vi "Find Invalid Plugin Groups by ID.vi"(8 "error in (no error)":errorcluster, 10 "plugin ID":string, 11 "Configuration Session in":refnum<class "Configuration Session.lvclass">) -> (0 "error out":errorcluster, 1 "Invalid Groups":string[](array[string]), 3 "Configuration Session out":refnum<class "Configuration Session.lvclass">, 4 "found?":bool)   [LabVIEW 2017, in "DSF Core.lvlib" / "Configuration Session.lvclass"]
uses:
  Configuration Session.lvclass
  Read Plugin Group IDs.vi
  Read All Group IDs.vi
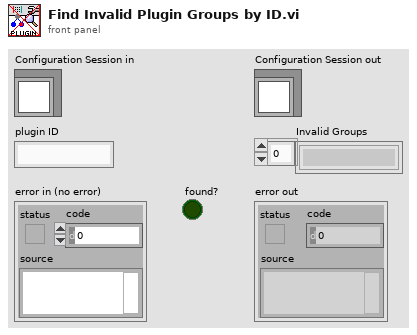
[diagram p1: front panel]
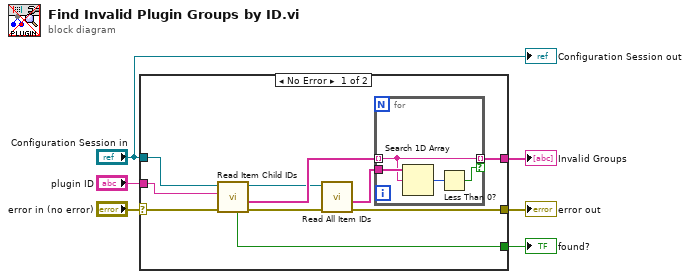
[diagram p0: block diagram]
diagram:
  n1 = case shown="No Error" "error in (no error)" {
    selector: "error in (no error)" -> [w14 w21]
    tunnel: "Configuration Session in" -> [w13 _]
    tunnel: [w8 w21] -> w4
    tunnel: "plugin ID" -> [w16 _]
    tunnel: [w15 _] -> w2
    tunnel: [w10 _] -> w1
    frame No Error {
      n2 = call-poly "Read Item Child IDs.vi"("error in (no error)"=w14, "Plugin ID"=w16, "Configuration Session"=w13) -> ("error out"=w9:errorcluster, "Group IDs"=w12:string[], "Configuration Session out"=w7:refnum<class "Configuration Session.lvclass">, "found?"=w15:bool)  [unwired: 5 in]
      n3 = call-poly "Read All Item IDs.vi"("error in (no error)"=w9, "Configuration Session in"=w7) -> ("error out"=w8:errorcluster, "Group IDs"=w11:string[])  [unwired: 7 in, 1 out]
      n4 = for {
        tunnel: w12 -> [w18] mode=indexing
        tunnel: w11 -> [w20]
        tunnel: [w18] -> w10 mode=indexing if=w17
        n5 = Search 1D Array(1D array=w20, element=w18) -> (index of element=w19:i32)  [unwired: 1 in]
        n6 = Less Than 0?(x=w19) -> (x < 0?=w17:bool)
      }
    }
    frame Error {
    }
  }
  "error out" <- w4
  "found?" <- w2
  "Invalid Groups" <- w1
  "Configuration Session out" <- "Configuration Session in"
